vi "TDMSAdv getData.vi"(5 "channel name":string, 6 "stringSplit? (T)":bool=TRUE, 7 "group name":string, 8 "error in (no error)":errorcluster, 11 "tdms1.0 file":refnum<k34>) -> (0 "error out":errorcluster, 2 "dataArr":string[](array[string]), 3 "tdms1.0 file out":refnum<k34>)   [LabVIEW 2018, in "TDMSAdv.lvclass"]
uses:
  TDMSAdv.lvclass
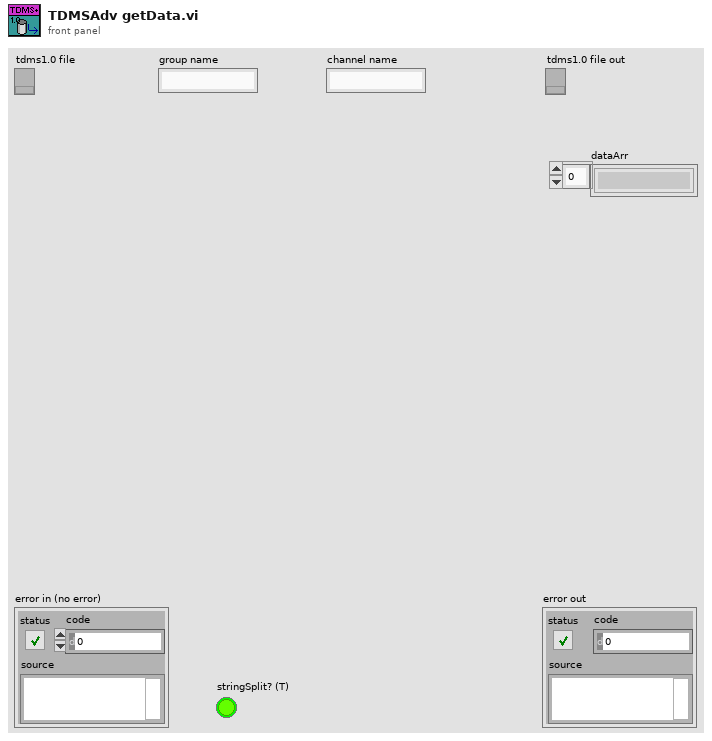
[diagram p1: front panel]
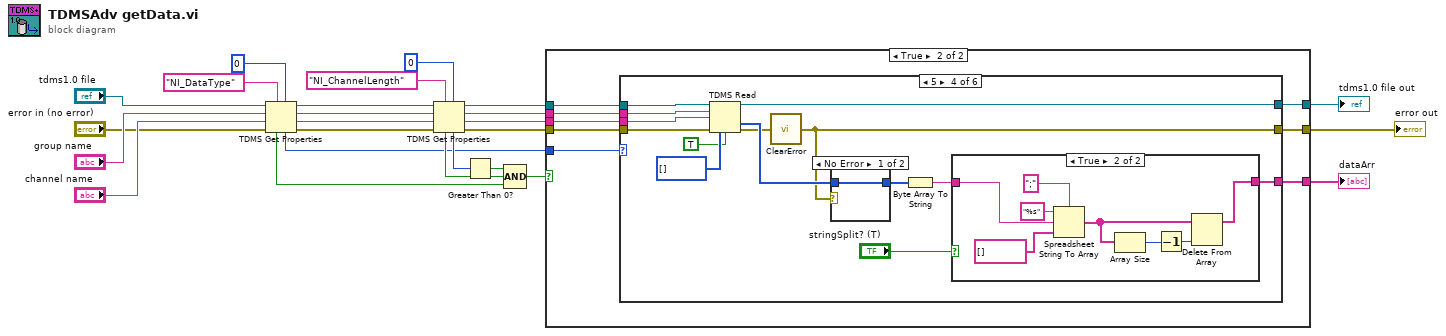
[diagram p0: block diagram]
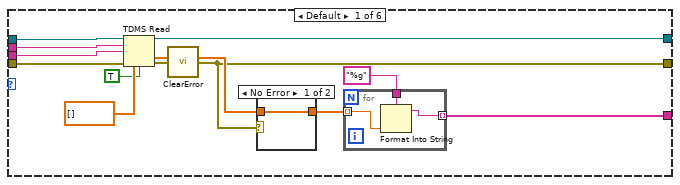
[diagram p3: hidden frame]
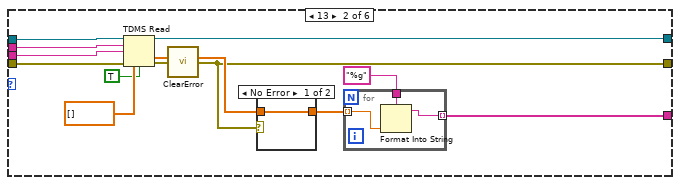
[diagram p5: hidden frame]
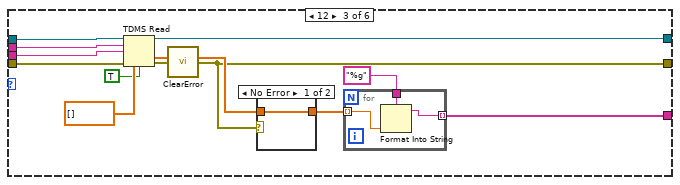
[diagram p7: hidden frame]
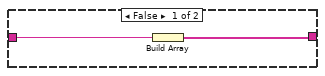
[diagram p9: hidden frame]
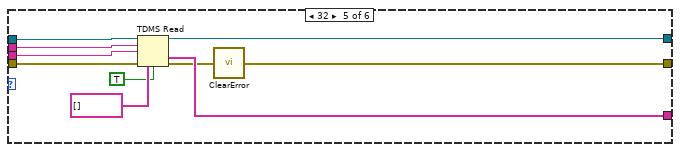
[diagram p11: hidden frame]
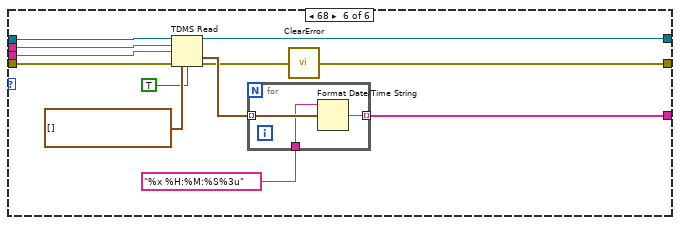
[diagram p12: hidden frame]
diagram:
  n1 = TDMS Get Properties(5:u16 0, 7:"NI_DataType" ("property name"), 8:"error in (no error)", 9:"channel name", 10:"group name", 11:"tdms1.0 file") -> (0:w23:errorcluster, 1:w20:string, 2:w21:string, 3:w22:refnum<k34>, 4:w8:u16, 6:w11:bool)
  n2 = TDMS Get Properties(5:u64 0, 7:"NI_ChannelLength" ("property name"), 8:w23, 9:w20, 10:w21, 11:w22) -> (0:w14:errorcluster, 1:w15:string, 2:w16:string, 3:w17:refnum<k34>, 4:w9:u64, 6:w10:bool)
  n3 = Greater Than 0?(x=w9) -> (x > 0?=w13:bool)
  n4 = Compound Arithmetic op=AND(w13, w10, w11) -> (w12:bool)
  n5 = case shown="True" w12 {
    tunnel: [w27 w30] -> w2
    tunnel: w17 -> [w26 w35]
    tunnel: w14 -> [w27 w34]
    tunnel: w16 -> [_ w33]
    tunnel: w15 -> [_ w32]
    tunnel: w8 -> [_ w31]
    tunnel: [_ w29] -> w1
    tunnel: [w26 w28] -> w3
    frame False {
    }
    frame True {
      n6 = case shown="5" w31 {
        tunnel: [w46 w63 w80 w98 w116 w133] -> w30
        tunnel: [w42 w59 w76 w88 w115 w132] -> w29
        tunnel: w35 -> [w37 w54 w71 w92 w121 w127]
        tunnel: w34 -> [w40 w57 w74 w95 w118 w124]
        tunnel: w33 -> [w38 w55 w72 w93 w120 w126]
        tunnel: w32 -> [w39 w56 w73 w94 w119 w125]
        tunnel: [w36 w53 w70 w89 w112 w122] -> w28
        frame Default {
          n7 = TDMS Read(0:w37, 5:w38, 7:w39, 11:w40, 12:dbl[] [], 13:TRUE ("return channels in file order? (F)")) -> (4:w36:refnum<k34>, 10:w48:dbl[], 15:w45:errorcluster)  [unwired: 2 in, 3 out]
          n8 = call <vilib>:"ClearError.vi"("error in (no error)"=w45) -> ("error out"=w46:errorcluster)
          n9 = case shown="No Error" w46 {
            tunnel: w48 -> [w52 _]
            tunnel: [w52 _] -> w43
            frame No Error {
            }
            frame Error {
            }
          }
          n10 = for {
            tunnel: "%g" ("format string") -> [w51]
            tunnel: w43 -> [w50] mode=indexing
            tunnel: [w49] -> w42 mode=indexing
            n11 = Format Into String(format string=w51, w50) -> (resulting string=w49:string)  [unwired: 2 in, 1 out]
          }
        }
        frame 13 {
          n12 = TDMS Read(0:w54, 5:w55, 7:w56, 11:w57, 12:dbl[] [], 13:TRUE ("return channels in file order? (F)")) -> (4:w53:refnum<k34>, 10:w65:dbl[], 15:w62:errorcluster)  [unwired: 2 in, 3 out]
          n13 = call <vilib>:"ClearError.vi"("error in (no error)"=w62) -> ("error out"=w63:errorcluster)
          n14 = case shown="No Error" w63 {
            tunnel: w65 -> [w69 _]
            tunnel: [w69 _] -> w60
            frame No Error {
            }
            frame Error {
            }
          }
          n15 = for {
            tunnel: "%g" ("format string") -> [w68]
            tunnel: w60 -> [w67] mode=indexing
            tunnel: [w66] -> w59 mode=indexing
            n16 = Format Into String(format string=w68, w67) -> (resulting string=w66:string)  [unwired: 2 in, 1 out]
          }
        }
        frame 12 {
          n17 = TDMS Read(0:w71, 5:w72, 7:w73, 11:w74, 12:sgl[] [], 13:TRUE ("return channels in file order? (F)")) -> (4:w70:refnum<k34>, 10:w82:sgl[], 15:w79:errorcluster)  [unwired: 2 in, 3 out]
          n18 = call <vilib>:"ClearError.vi"("error in (no error)"=w79) -> ("error out"=w80:errorcluster)
          n19 = case shown="No Error" w80 {
            tunnel: w82 -> [w86 _]
            tunnel: [w86 _] -> w77
            frame No Error {
            }
            frame Error {
            }
          }
          n20 = for {
            tunnel: "%g" ("format string") -> [w85]
            tunnel: w77 -> [w84] mode=indexing
            tunnel: [w83] -> w76 mode=indexing
            n21 = Format Into String(format string=w85, w84) -> (resulting string=w83:string)  [unwired: 2 in, 1 out]
          }
        }
        frame 5 {
          n22 = TDMS Read(0:w92, 5:w93, 7:w94, 11:w95, 12:u8[] [], 13:TRUE ("return channels in file order? (F)")) -> (4:w89:refnum<k34>, 10:w100:u8[], 15:w97:errorcluster)  [unwired: 2 in, 3 out]
          n23 = call <vilib>:"ClearError.vi"("error in (no error)"=w97) -> ("error out"=w98:errorcluster)
          n24 = case shown="No Error" w98 {
            tunnel: w100 -> [w111 _]
            tunnel: [w111 _] -> w91
            frame No Error {
            }
            frame Error {
            }
          }
          n25 = Byte Array To String(unsigned byte array=w91) -> (string=w90:string)
          n26 = case shown="True" "stringSplit? (T)" {
            tunnel: w90 -> [w102 w109]
            tunnel: [w101 w103] -> w88
            frame False {
              n27 = Build Array(w102) -> (w101:string[])
            }
            frame True {
              n28 = Spreadsheet String To Array(delimiter (Tab)=";", format string="%s", spreadsheet string=w109, array type (2D Dbl)=string[] []) -> (array=w106:string[])
              n29 = Array Size(array=w106) -> (size(s)=w105:i32)
              n30 = Decrement(x=w105) -> (x-1=w104:i32)
              n31 = Delete From Array(array=w106, index=w104) -> (array with subset deleted=w103:string[])  [unwired: 1 in, 1 out]
            }
          }
        }
        frame 32 {
          n32 = TDMS Read(0:w121, 5:w120, 7:w119, 11:w118, 12:string[] [], 13:TRUE ("return channels in file order? (F)")) -> (4:w112:refnum<k34>, 10:w115:string[], 15:w114:errorcluster)  [unwired: 2 in, 3 out]
          n33 = call <vilib>:"ClearError.vi"("error in (no error)"=w114) -> ("error out"=w116:errorcluster)
        }
        frame 68 {
          n34 = TDMS Read(0:w127, 5:w126, 7:w125, 11:w124, 12:timestamp[] [], 13:TRUE ("return channels in file order? (F)")) -> (4:w122:refnum<k34>, 10:w131:timestamp[], 15:w130:errorcluster)  [unwired: 2 in, 3 out]
          n35 = for {
            tunnel: [w136] -> w132 mode=indexing
            tunnel: w131 -> [w135] mode=indexing
            tunnel: "%x %H:%M:%S%3u" ("time format string (%c)") -> [w134]
            n36 = Format Date/Time String(time format string (%c)=w134, seconds (now)=w135) -> (date/time string=w136:string)  [unwired: 1 in]
          }
          n37 = call <vilib>:"ClearError.vi"("error in (no error)"=w130) -> ("error out"=w133:errorcluster)
        }
      }
    }
  }
  "tdms1.0 file out" <- w3
  "error out" <- w2
  "dataArr" <- w1
